vi "LVClass_ModalCoef SetLegendrePrefs.vi"(0 "ModalCoef in":refnum<class "ModalCoef.lvclass">, 5 "LegendreModalPrefs":T1={"Number of coefficients"=32, "Filtered coefficients"=[], "RMS Legendre normalization"=FALSE, "RectangularProjectionPupilDimensions"={"Pupil center_sspp"={"X"=0.0, "Y"=0.0}, "Pupil halfsize_sspp"={"X"=0.0, "Y"=0.0}}}, 11 "error in (no error)":errorcluster) -> (4 "ModalCoef out":refnum<class "ModalCoef.lvclass">, 15 "error out":errorcluster)   [LabVIEW 2020, in "ModalCoef.lvclass"]
doc: "Set the Legendre preferences for modal phase reconstruction.\n\n--------------------------------------------------------------------------------\n\n<B>ComputePhaseSetIn </B> : ComputePhaseSet object.\n<B>ComputePhaseSetOut </B> : ComputePhaseSet object.\n<B>nb_coeffs_total </B> : Number of the Legendre coefficients used in the polynomial base.\n<B>nb_coeffs_to_filter </B> : Number of the Legendre coefficients to filter in the polynomial base.\n<B>coeffs_to_filter </B> : List of indices of the Legendre coefficients to filter in the polynomial base.\n<B>projection_pupil_center </B> : Center of the projection pupil, in number of subpupils.\n<B>projection_pupil_halfsize </B> : Projection pupil half size, in number of subpupils.\n<B>ErrorIn </B> : Error\n<B>ErrorOut </B> : Error\n\n--------------------------------------------------------------------------------"
uses:
  ModalCoef.lvclass
  LegendreModalPrefs.ctl
  LegendreProjectionPupilSetup.ctl
  Point2Df.ctl
  ModalCoef.lvclass/ModalCoef.ctl
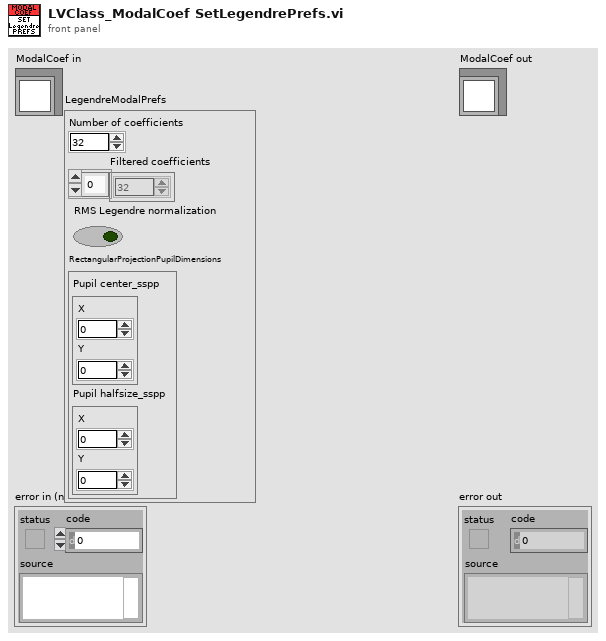
[diagram p1: front panel]
types:
  T1 = typedef "LegendreModalPrefs.ctl" = cluster{"Number of coefficients":u32, "Filtered coefficients":u32[], "RMS Legendre normalization":bool, "RectangularProjectionPupilDimensions":T2}
  T2 = typedef "LegendreProjectionPupilSetup.ctl" = cluster{"Pupil center_sspp":T3, "Pupil halfsize_sspp":T3}
  T3 = typedef "Point2Df.ctl" = cluster{"X":sgl, "Y":sgl}
  T4 = typedef "ClassID.ctl" = i64
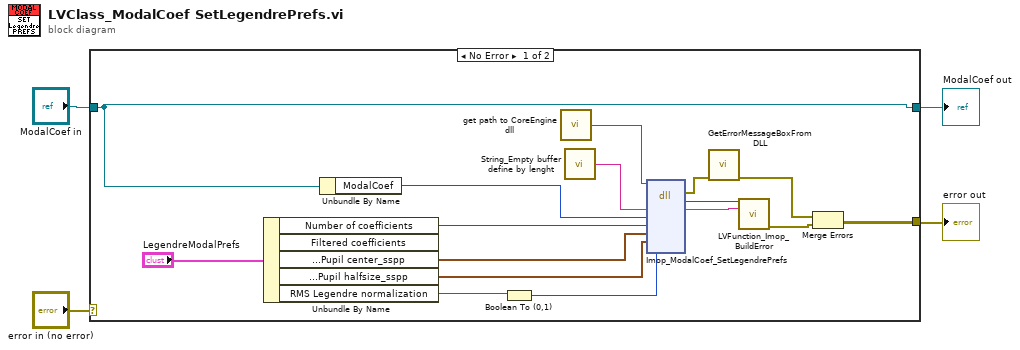
[diagram p0: block diagram]
diagram:
  n1 = case shown="No Error" "error in (no error)" {
    selector: "error in (no error)" -> [_ w22]
    tunnel: [w7 w22] -> w1
    tunnel: [w11 w21] -> w3
    tunnel: "ModalCoef in" -> [w11 w21]
    frame No Error {
      n2 = Unbundle By Name("LegendreModalPrefs") -> ("Number of coefficients"=w14:u32, "RectangularProjectionPupilDimensions.Pupil center_sspp"=w13:T3, "RectangularProjectionPupilDimensions.Pupil halfsize_sspp"=w12:T3, "RMS Legendre normalization"=w6:bool)  [unwired: 1 out]
      n3 = Unbundle By Name(w11) -> ("ModalCoef"=w10:T4)
      n4 = Boolean To (0,1)(Boolean=w6) -> (0, 1=w5:i16)
      n5 = call "get path to CoreEngine dll.vi"() -> ("path to wavekit library"=w17:path)  [unwired: 14 in, 1 out]
      n6 = call "String_Empty buffer define by lenght.vi"() -> ("Empty buffer"=w18:string)  [unwired: 1 in]
      n7 = dll-call lib="D:/2_trunk/Soft_haso/ImOpCoreEngine4_LV2011/DLLs/ImopEngine4_vc100.dll" fn="Imop_ModalCoef_SetLegendrePrefs"(path in=w17, "message"=w18, "objet"=w10, "numberOfCoefficient"=w14, "projection_pupil_center"=w13, "projection_pupil_size"=w12, "normalization"=w5) -> (error out=w16:errorcluster, "return type"=w20:i32, "message"=w19:string)  [unwired: 7 in, 1 out]
      n8 = call "GetErrorMessageBoxFromDLL.vi"("error IN"=w16) -> ("error OUT"=w9:errorcluster)  [unwired: 10 in]
      n9 = call "LVFunction_Imop_BuildError.vi"("code"=w20, "String to Prepend to source (\"\")"=w19) -> ("error out"=w8:errorcluster)  [unwired: 13 in]
      n10 = Merge Errors(w9, w8) -> (w7:errorcluster)
    }
    frame Error {
    }
  }
  "error out" <- w1
  "ModalCoef out" <- w3
